vi "IR.vi"() -> ()   [LabVIEW 2015]
panel:
  in  "?":bool
  out "?":dbl(knob) scale=0.0..50.0
  # "DISTANCE"
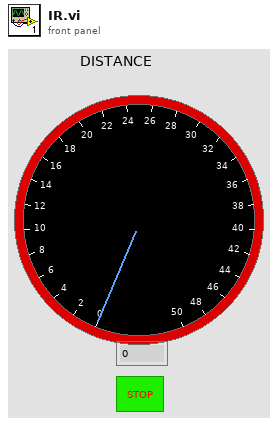
[diagram p1: front panel]
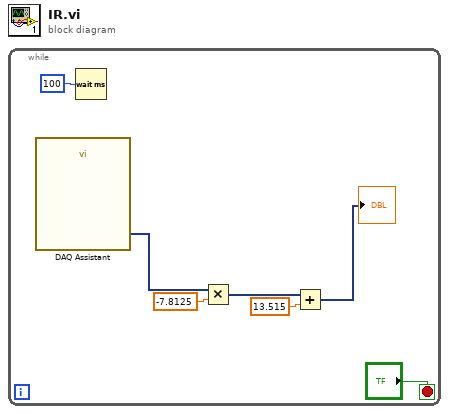
[diagram p0: block diagram]
diagram:
  n1 = while {
    stop <- "?" stop-if-true
    n2 = call "DAQ Assistant"() -> ("data"=w7:dynamicdata)  [unwired: 17 in, 2 out]
    n3 = Wait (ms)(milliseconds to wait=u32 100) -> ()  [unwired: 1 out]
    n4 = Multiply(x=w7, y=-7.8125) -> (x*y=w5:dynamicdata)
    n5 = Add(x=w5, y=13.515) -> (x+y=→"?":dynamicdata)
  }
